vi "PID Set Profiled.vi"(10 "Profiled?":bool, 11 "PID Ref":refnum<data-value>) -> (3 "PID Ref":refnum<data-value>)   [LabVIEW 2019]
uses:
  Typedef/PID Controller State.ctl
panel:
  # "NOTE: Currently this is not bumpless\n\nTODO: Add initial condition on change from non-profiled --> profiled"
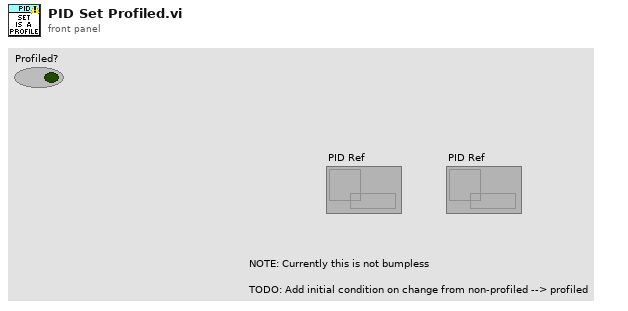
[diagram p1: front panel]
types:
  T1 = typedef "PID Controller State.ctl" = cluster{"PIDF Gains":cluster{"Kp":dbl, "Ki":dbl, "Kd":dbl, "Kf":dbl}, "Output Range":cluster{"output high":dbl, "output low":dbl}, "Profiled?":bool, "PID State":cluster{"iState":dbl, "dState":dbl, "Error [n-1]":dbl, "Output":dbl}, "Setpoint":dbl, "Profiled State":cluster{"Position":dbl, "Velocity":dbl}, "Profiled Contraints":cluster{"Max Velocity":dbl, "Max Acceleration":dbl}}
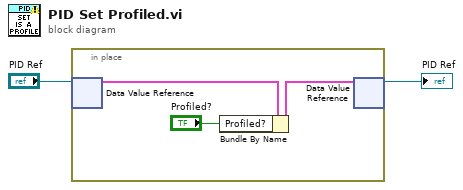
[diagram p0: block diagram]
diagram:
  n1 = in-place {
    n2 = in-place-dvr #1("PID Ref") -> (w5:T1)  [unwired: 1 out]
    n3 = Bundle By Name(cluster=w5, "Profiled?"="Profiled?") -> (w4:T1)
    n4 = in-place-dvr #1(w4) -> (→"PID Ref":refnum<data-value>)  [unwired: 1 out]
  }
